vi "TSLIN Transmit.vi"(0 "路径输入":path, 11 "错误输入（无错误）":errorcluster, 12 "TLIN":T1 {"AIdxChn" items=["CHN1", "CHN2", "CHN3", "CHN4", "CHN5", "CHN6", "CHN7", "CHN8", "CHN9", "CHN10", "CHN11", "CHN12", "CHN13", "CHN14", "CHN15", "CHN16", "CHN17", "CHN18", "CHN19", "CHN20", "CHN21", "CHN22", "CHN23", "CHN24", "CHN25", "CHN26", "CHN27", "CHN28", "CHN29", "CHN30", "CHN31", "CHN32"]}) -> (4 "路径输出":path, 15 "错误输出":errorcluster)   [LabVIEW 2013]
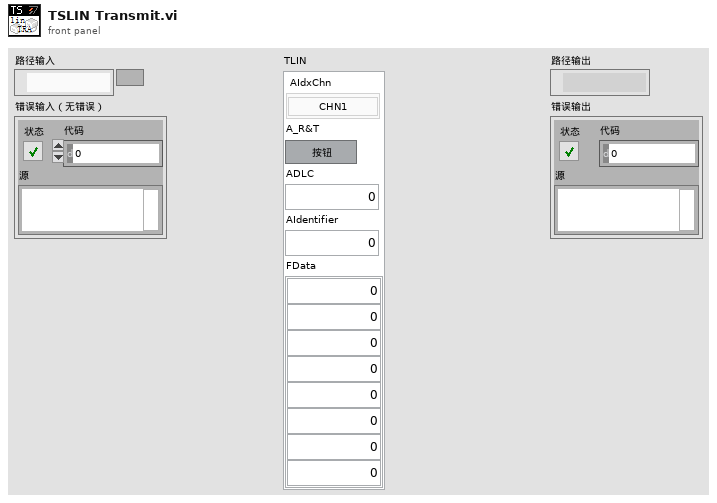
[diagram p1: front panel]
types:
  T1 = cluster{"AIdxChn":u8, "A_R&T":bool, "ADLC":u8, "AIdentifier":u8, "FData":cluster{"Data 0":u8, "Data 1":u8, "Data 2":u8, "Data 3":u8, "Data 4":u8, "Data 5":u8, "Data 6":u8, "Data 7":u8}}
  T2 = cluster{"FidxChn":u8, "FErrStatus":u8, "FProperties":u8, "FDLC":u8, "FIdentifier":u8, "FChecksum":u16, "FtimeUS":u64, "FData":cluster{"Data 0":u8, "Data 1":u8, "Data 2":u8, "Data 3":u8, "Data 4":u8, "Data 5":u8, "Data 6":u8, "Data 7":u8}}
  T3 = cluster{"Data 0":u8, "Data 1":u8, "Data 2":u8, "Data 3":u8, "Data 4":u8, "Data 5":u8, "Data 6":u8, "Data 7":u8}
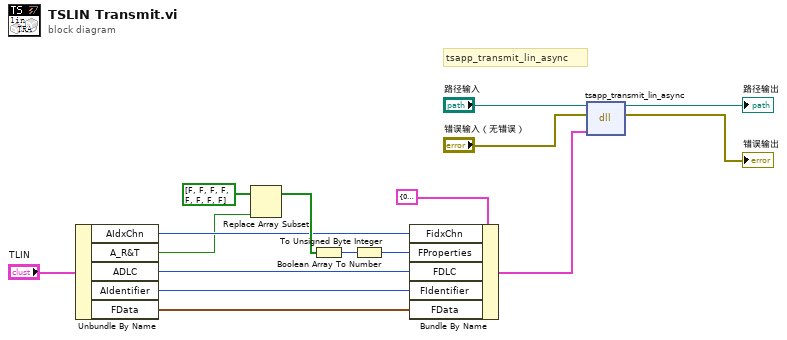
[diagram p0: block diagram]
diagram:
  # "tsapp_transmit_lin_async"
  n1 = Unbundle By Name("TLIN") -> ("AIdxChn"=w5:u8, "A_R&T"=w4:bool, "ADLC"=w3:u8, "AIdentifier"=w2:u8, "FData"=w1:T3)
  n2 = Replace Array Subset(array=bool[] [FALSE, FALSE, FALSE, FALSE, FALSE, FALSE, FALSE, FALSE], new element=w4) -> (w7:bool[])  [unwired: 1 in]
  n3 = Boolean Array To Number(Boolean array=w7) -> (number=w12:u32)
  n4 = To Unsigned Byte Integer(number=w12) -> (unsigned 8bit integer=w11:u8)
  n5 = Bundle By Name(cluster=T2 {"FidxChn"=0, "FErrStatus"=0, "FProperties"=0, "FDLC"=0, "FIdentifier"=0, "FChecksum"=0, "FtimeUS"=0, "FData"={"Data 0"=0, "Data 1"=0, "Data 2"=0, "Data 3"=0, "Data 4"=0, "Data 5"=0, "Data 6"=0, "Data 7"=0}} ("TLIBIN"), "FidxChn"=w5, "FProperties"=w11, "FDLC"=w3, "FIdentifier"=w2, "FData"=w1) -> (w10:T2)
  n6 = dll-call lib="PTH1@abs EDemo同星TSCAN_V1.4_20220301ConfigTSMaster.dll" fn="tsapp_transmit_lin_async"(path in="路径输入", error in="错误输入（无错误）", "LINDATA"=w10) -> (path out=→"路径输出":path, error out=→"错误输出":errorcluster)  [unwired: 3 in]
